vi "Excel Read.vi"(8 "error in (no error)":errorcluster, 9 "end (-1, -1)":cluster{"row":i32, "column":i32}={"row"=-1, "column"=-1}, 10 "start (-1, -1)":cluster{"row":i32, "column":i32}={"row"=-1, "column"=-1}, 11 "template (empty)":path) -> (0 "error out":errorcluster, 3 "Array":string[][](array[string]))   [LabVIEW 2021]
uses:
  <vilib>/Utility/NIReport.llb/Report Type.ctl
  <vilib>/addons/_office/excel.llb/Excel Get Data ([str]).vi
  <vilib>/Utility/NIReport.llb/NI_report.lvclass
  <vilib>/addons/_office/NI_ReportGenerationToolkit.lvlib
  <vilib>/Utility/NIReport.llb/Excel/NI_Excel.lvclass
  <vilib>/Utility/NIReport.llb/NI_ReportGenerationCore.lvlib
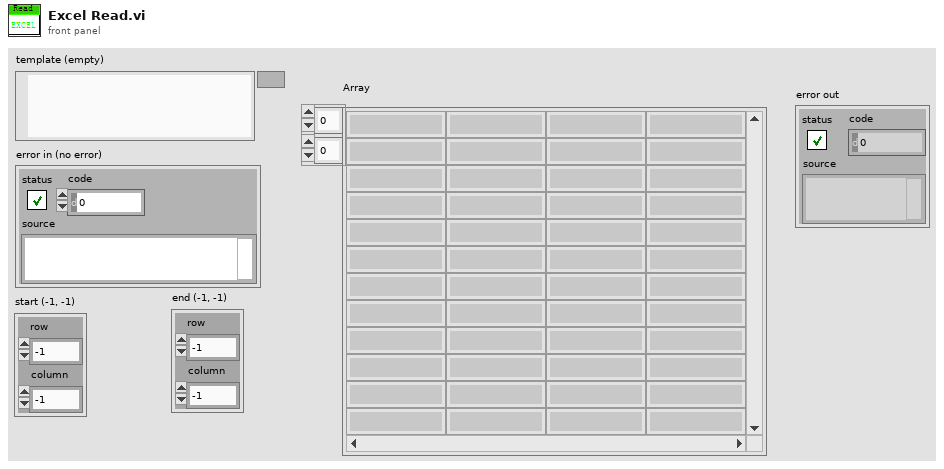
[diagram p1: front panel]
types:
  T1 = typedef "NI_ReportGenerationCore.lvlib/Report Type.ctl" = enum16{"HTML", "Word", "Excel"}
  T2 = enum16{"maximized", "minimized", "normal", "no change"}
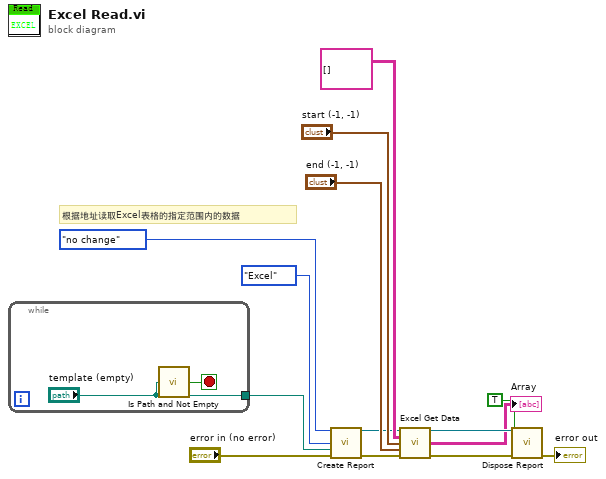
[diagram p0: block diagram]
diagram:
  # "根据地址读取Excel表格的指定范围内的数据"
  n1 = while {
    tunnel: ["template (empty)"] -> w6
    stop <- w15 stop-if-true
    n2 = call <vilib>:"Is Path and Not Empty.vi"("path"="template (empty)") -> ("Is Path and Not Empty?"=w15:bool)  [unwired: 4 in]
  }
  n3 = call <vilib>:"Create Report.vi"("window state (normal)"=T2."no change", "report type"=Report_Type."Excel", "template (empty)"=w6, "error in (no error)"="error in (no error)") -> ("report out"=w4:refnum<class "NI_report.lvclass">, "error out"=w3:errorcluster)  [unwired: 10 in]
  n4 = call-poly <vilib>:"Excel Get Data.vi"("report in"=w4, "data type"=string[][] [] ("Array 2"), "start (-1, -1)"="start (-1, -1)", "end (-1, -1)"="end (-1, -1)", "error in (no error)"=w3) -> ("report out"=w14:refnum<class "NI_report.lvclass">, "data"=→"Array":string[][], "error out"=w13:errorcluster)  [unwired: 8 in]
  n5 = call-dynamic "Dispose Report.vi"("report in"=w14, "save changes? (F)"=TRUE, "error in (no error)"=w13) -> ("error out"=→"error out":errorcluster)  [unwired: 12 in]
